vi "Configure System.vi"(6 "Line Frequency (0: 50 Hz)":u16(ring) items=["50 Hz", "60 Hz"], 8 "error in (no error)":errorcluster, 9 "Guard (0: Internal)":u16(ring) items=["Internal", "External"], 10 "Terminals (0: Front)":u16(ring) items=["Front", "Rear", "Ratio", "Difference", "Deviation", "OFF"], 11 "VISA resource name":refnum<visa-resource-name>) -> (0 "error out":errorcluster, 3 "VISA resource name out":refnum<visa-resource-name>)   [LabVIEW 2012, in "Fluke 8508.lvlib"]
doc: "This VI configures system settings on the instrument such as the terminals (normal or scan), function guarding and line frequency."
uses:
  Fluke 8508.lvlib
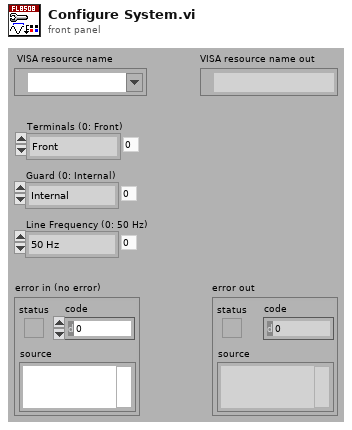
[diagram p1: front panel]
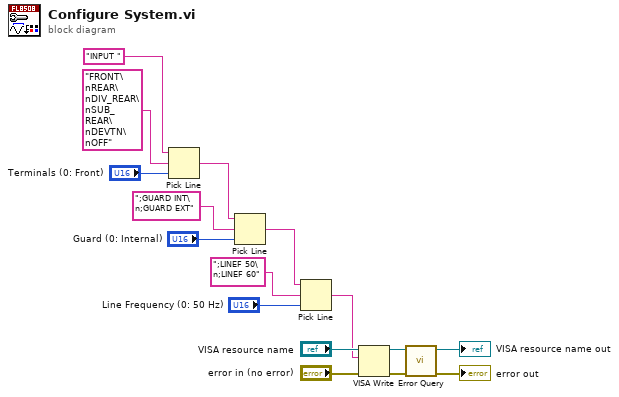
[diagram p0: block diagram]
diagram:
  n1 = Pick Line(string ("")="INPUT ", multi-line string="FRONT\nREAR\nDIV_REAR\nSUB_REAR\nDEVTN\nOFF", line index="Terminals (0: Front)") -> (output string=w6:string)
  n2 = Pick Line(string ("")=w6, multi-line string=";GUARD INT\n;GUARD EXT", line index="Guard (0: Internal)") -> (output string=w5:string)
  n3 = Pick Line(string ("")=w5, multi-line string=";LINEF 50\n;LINEF 60", line index="Line Frequency (0: 50 Hz)") -> (output string=w2:string)
  n4 = VISA Write(VISA resource name="VISA resource name", write buffer=w2, error in (no error)="error in (no error)") -> (VISA resource name out=w12:refnum<visa-resource-name>, error out=w11:errorcluster)  [unwired: 1 out]
  n5 = call "Error Query.vi"("error in (no error)"=w11, "VISA resource name"=w12) -> ("error out"=→"error out":errorcluster, "VISA resource name out"=→"VISA resource name out":refnum<visa-resource-name>)  [unwired: 6 in, 2 out]
